vi "3.8-Create Midbrain Neuron.vi"() -> (0 "data string":string)   [LabVIEW 2010]
uses:
  6-OCU Neurons/6.3-Lidar Data.ctl
  4-High Neurons/4.8-Midbrain to Forebrain Neuron.ctl
  4-High Neurons/4.2-Where Sensor Typedef.ctl
  4-High Neurons/Current GPS Data.ctl
  3.2-Where/_typedefs/3.2.1-VectorNav Data.ctl
  4-High Neurons/4.1-Midbrain Act Data.ctl
  4-High Neurons/4.4-How Sensor Typedef.ctl
  4-High Neurons/4.0-Midbrain State.ctl
  4-High Neurons/4.2/4.2.0 Kalman State.ctl
  3.0-Global.vi
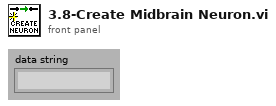
[diagram p1: front panel]
types:
  T1 = enum16{"Set Midbrain Act Data", "Read Midbrain Act Data"}
  T2 = typedef "4.8-Midbrain to Forebrain Neuron.ctl" = cluster{"6.7-Lidar Data":T3, "4.2-Where Am I? Sensor":T4, "4.1- Midbrain Act Data":T7, "4.4-How Am I? Sensor":T8, "3.2.0 State Vector X":T10}
  T3 = typedef "6.3-Lidar Data.ctl" = cluster{"Angle Array":dbl[], "Magnitude Array":dbl[]}
  T4 = typedef "4.2-Where Sensor Typedef.ctl" = cluster{"4.2.2- Current GPS Data":T5, "4.2.1-VectorNav Data":T6, "4.2.1-VectorNav Status":string}
  T5 = typedef "Current GPS Data.ctl" = cluster{"Lattitude (Decimal Degrees)":ext, "Longitude (Decimal Degrees)":ext, "EST Time":timestamp}
  T6 = typedef "3.2.1-VectorNav Data.ctl" = cluster{"Yaw":dbl, "Pitch":dbl, "Roll":dbl}
  T7 = typedef "4.1-Midbrain Act Data.ctl" = cluster{"Arbitrated Array":sgl[], "Exploded Obstacles":sgl[], "Desired Change in Heading":sgl, "Desired Speed Fraction":sgl}
  T8 = typedef "4.4-How Sensor Typedef.ctl" = cluster{"Motor Speed Integer":i32, "Drive Position Integer":i32, "Lidar Position Integer":i32, "Lidar Motor Position Integer":i32, "Steering Position Integer":i32, "Battery Voltage Fxp":dbl, "Drive Encoder Cable Check":bool, "Lidar Drive Encoder Cable Check":bool, "Steer Encoder Cable Check":bool, "Lidar Pos Encoder Cable Check":bool, "Mod Buttons & Blinky Cable Check":bool, "Lidar Data Cable Check":bool, "Drive Motor Cable Check":bool, "Vector Nav Cable Check":bool, "Lidar Drive Cable Check":bool, "Steer Drive Cable Check":bool, "Reverse?":bool, "2.1  Steering Control Voltage":dbl, "2.1 Drive Control Voltage":dbl, "2.1  Lidar Control Voltage":dbl, "2.5.7 A*B":dbl, "2.1  Steering PID Output":dbl, "2.1 Drive PID Output":dbl, "2.1  Lidar PID Output":dbl, "2.1.1 Drive Error":dbl, "2.1.1 Drive Error I":dbl, "2.1.1 Drive Error D":dbl, "2.1.2 Steering Error":dbl, "2.1.2 Steering Error I":dbl, "2.1.2 Steering Error D":dbl, "2.1.3 Lidar Error":dbl, "2.1.3 Lidar Error I":dbl, "2.1.3 Lidar Error D":dbl, "VectorNav Ack Query":bool, "VectorNav Read Byte":u8, "VectorNav Read Status":enum16{"Waiting", "Reading", "Done"}, "4.0-Midbrain State":T9}
  T9 = typedef "4.0-Midbrain State.ctl" = enum16{"Startup", "Waiting to Run", "Running-OlinOval", "Running-ChannelFollow", "Running-WallFollow", "Running-OpenTransit", "Running-Joystick Training", "Shutdown", "Restart"}
  T10 = typedef "4.2.0 Kalman State.ctl" = cluster{"X":dbl, "Y":dbl, "Theta":dbl, "V":dbl, "Omega":dbl, "Omega Dot":dbl}
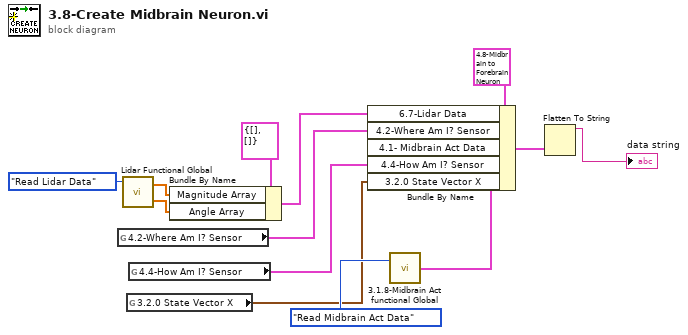
[diagram p0: block diagram]
diagram:
  n1 = global read "3.0-Global.vi" "4.2-Where Am I? Sensor"() -> (w5:T4)
  n2 = call "Lidar Functional Global.vi"("Lidar Action"=enum16{"Set Lidar Data", "Read Lidar Data"}."Read Lidar Data") -> ("Lidar Angle Data Out (Degrees)"=w13:sgl[], "Lidar Magnitude Data Out (mm)"=w12:sgl[])  [unwired: 2 in]
  n3 = global read "3.0-Global.vi" "3.2.0 State Vector X"() -> (w1:T10)
  n4 = global read "3.0-Global.vi" "4.4-How Am I? Sensor"() -> (w2:T8)
  n5 = Bundle By Name(cluster=T3 {"Angle Array"=[], "Magnitude Array"=[]} ("6.7-Lidar Data"), "Magnitude Array"=w12, "Angle Array"=w13) -> (w7:T3)
  n6 = call "3.1.8-Midbrain Act functional Global.vi"("Command"=T1."Read Midbrain Act Data") -> ("4.1- Outputted Midbrain Act Data"=w3:T7)  [unwired: 1 in]
  n7 = Bundle By Name(cluster=T2 {"6.7-Lidar Data"={"Angle Array"=[], "Magnitude Array"=[]}, "4.2-Where Am I? Sensor"={"4.2.2- Current GPS Data"={"Lattitude (Decimal Degrees)"=0.0, "Longitude (Decimal Degrees)"=0.0, "EST Time"=timestamp(0 s since 1904-01-01)}, "4.2.1-VectorNav Data"={"Yaw"=0.0, "Pitch"=0.0, "Roll"=0.0}, "4.2.1-VectorNav Status"=""}, "4.1- Midbrain Act Data"={"Arbitrated Array"=[], "Exploded Obstacles"=[], "Desired Change in Heading"=0.0, "Desired Speed Fraction"=0.0}, "4.4-How Am I? Sensor"={"Motor Speed Integer"=0, "Drive Position Integer"=0, "Lidar Position Integer"=0, "Lidar Motor Position Integer"=0, "Steering Position Integer"=0, "Battery Voltage Fxp"=0.0, "Drive Encoder Cable Check"=FALSE, "Lidar Drive Encoder Cable Check"=FALSE, "Steer Encoder Cable Check"=FALSE, "Lidar Pos Encoder Cable Check"=FALSE, "Mod Buttons & Blinky Cable Check"=FALSE, "Lidar Data Cable Check"=FALSE, "Drive Motor Cable Check"=FALSE, "Vector Nav Cable Check"=FALSE, "Lidar Drive Cable Check"=FALSE, "Steer Drive Cable Check"=FALSE, "Reverse?"=FALSE, "2.1  Steering Control Voltage"=0.0, "2.1 Drive Control Voltage"=0.0, "2.1  Lidar Control Voltage"=0.0, "2.5.7 A*B"=0.0, "2.1  Steering PID Output"=0.0, "2.1 Drive PID Output"=0.0, "2.1  Lidar PID Output"=0.0, "2.1.1 Drive Error"=0.0, "2.1.1 Drive Error I"=0.0, "2.1.1 Drive Error D"=0.0, "2.1.2 Steering Error"=0.0, "2.1.2 Steering Error I"=0.0, "2.1.2 Steering Error D"=0.0, "2.1.3 Lidar Error"=0.0, "2.1.3 Lidar Error I"=0.0, "2.1.3 Lidar Error D"=0.0, "VectorNav Ack Query"=FALSE, "VectorNav Read Byte"=0, "VectorNav Read Status"=enum."Waiting", "4.0-Midbrain State"=enum."Startup"}, "3.2.0 State Vector X"={"X"=0.0, "Y"=0.0, "Theta"=0.0, "V"=0.0, "Omega"=0.0, "Omega Dot"=0.0}} ("4.8-Midbrain to Forebrain Neuron"), "6.7-Lidar Data"=w7, "4.2-Where Am I? Sensor"=w5, "4.1- Midbrain Act Data"=w3, "4.4-How Am I? Sensor"=w2, "3.2.0 State Vector X"=w1) -> (w6:T2)
  n8 = Flatten To String(anything=w6) -> (data string=→"data string":string)  [unwired: 3 in, 2 out]
